vi "Write T0.vi"(8 "error in (no error)":errorcluster, 10 "T0":ext, 11 "PmuBase in":refnum<class "PmuBase.lvclass">) -> (0 "error out":errorcluster, 3 "PmuBase out":refnum<class "PmuBase.lvclass">)   [LabVIEW 2014]
uses:
  PmuBase.lvclass
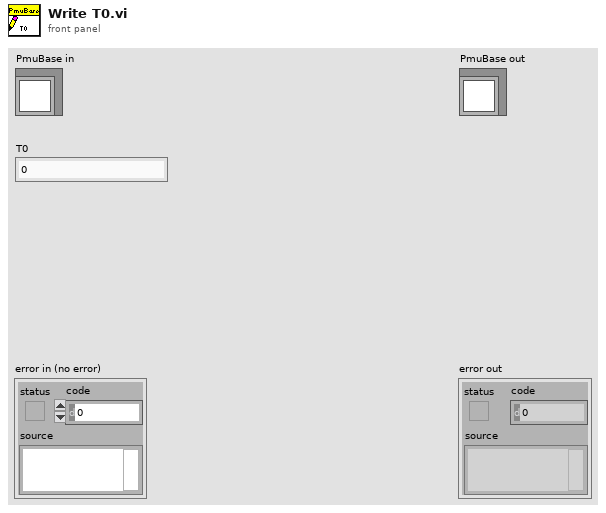
[diagram p1: front panel]
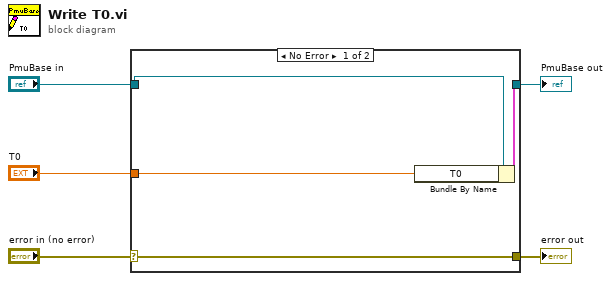
[diagram p0: block diagram]
diagram:
  n1 = case shown="No Error" "error in (no error)" {
    selector: "error in (no error)" -> [w9 w10]
    tunnel: [w9 w10] -> w4
    tunnel: [w7 w11] -> w2
    tunnel: "PmuBase in" -> [w8 w11]
    tunnel: "T0" -> [w6 _]
    frame No Error {
      n2 = Bundle By Name(cluster=w8, "T0"=w6) -> (w7:cluster{})
    }
    frame Error {
    }
  }
  "error out" <- w4
  "PmuBase out" <- w2
